vi "FILE.vi"   [LabVIEW 2016]
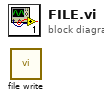
[diagram p0: block diagram]
diagram:
  n1 = call "file write.vi"() -> ()  [unwired: 2 in, 1 out]
